vi "integrate_phase.vi"(6 "integration method":T1=1 items=["Trapezoidal Rule", "Simpson's Rule", "Simpson's 3/8 Rule", "Bode Rule"], 9 "Integrand (function of wl) (units)":dbl[](array[numeric]), 11 "Wavelengths (ascending, evenly spaced) (nm)":dbl[](array[numeric])) -> (1 "Integral (function of wl) (10^15*units)":dbl[](array[numeric]))   [LabVIEW 2022 SP3]
uses:
  <vilib>/Analysis/2dsp.llb/Integral Method.ctl
  <vilib>/Analysis/8numeric.llb/1D Numeric Integration.vi
  <vilib>/Analysis/NI_AALPro.lvlib
panel:
  # "computes\n\\[ int_{\\omega_{min}}^\\omega  phase''(\\omega) \\, d\\omega \\]\nwith respect to \\lambda via substitution of \\omega = 2\\pi c / \\lambda"
  # "since phase'' is in fs^2 due to gamma^2 factor (check _MIIPS), as before we will use lambda in nm and c in Mm/s.\nThis way, integrating once gives 10^-15 s, and integrating again gives phase in radians."
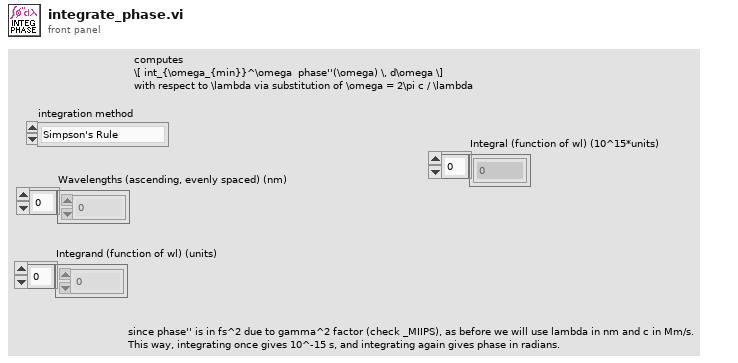
[diagram p1: front panel]
types:
  T1 = typedef "NI_AALPro.lvlib/Integral Method.ctl" = i32
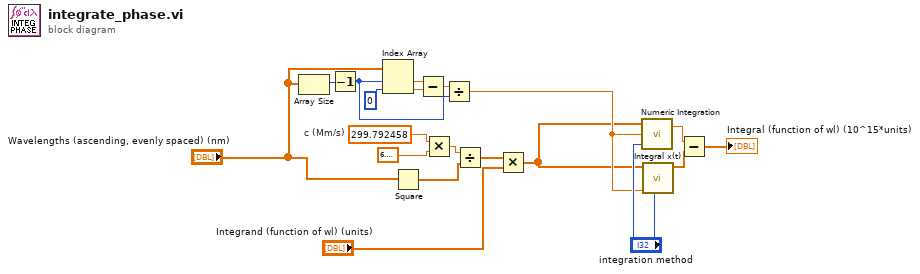
[diagram p0: block diagram]
diagram:
  w9 = 299.792458  # c (Mm/s)
  n1 = Array Size(array="Wavelengths (ascending, evenly spaced) (nm)") -> (size(s)=w12:i32)
  n2 = Decrement(x=w12) -> (x-1=w10:i32)
  n3 = Index Array(array="Wavelengths (ascending, evenly spaced) (nm)", index #1=w10, index #2=0) -> (element #1=w14:dbl, element #2=w15:dbl)
  n4 = Square(x="Wavelengths (ascending, evenly spaced) (nm)") -> (x^2=w5:dbl[])
  n5 = Subtract(x=w14, y=w15) -> (x-y=w13:dbl)
  n6 = Multiply(x=w9, y=6.283185307179586) -> (x*y=w6:dbl)
  n7 = Divide(x=w13, y=w10) -> (x/y=w11:dbl)
  n8 = Divide(x=w6, y=w5) -> (x/y=w2:dbl[])
  n9 = Multiply(x=w2, y="Integrand (function of wl) (units)") -> (x*y=w3:dbl[])
  n10 = call-poly <vilib>:"Numeric Integration.vi"("integration method"="integration method", "dt"=w11, "Input Array"=w3) -> ("result"=w18:dbl)  [unwired: 1 out]
  n11 = call <vilib>:"Integral x(t).vi"("integration method"="integration method", "dt"=w11, "X"=w3) -> ("Integral X"=w17:dbl[])  [unwired: 7 in, 1 out]
  n12 = Subtract(x=w18, y=w17) -> (x-y=→"Integral (function of wl) (10^15*units)":dbl[])
